vi "VolumetricFlow.vi"(9 "Pressure":dbl format="%#_13g", 10 "Tem":dbl format="%#_13g", 11 "Flow":dbl format="%#_13g") -> (3 "VolumetricFlow":dbl)   [LabVIEW 2017]
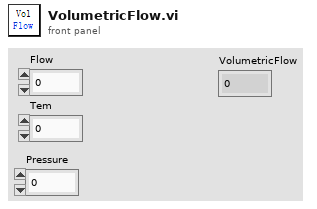
[diagram p1: front panel]
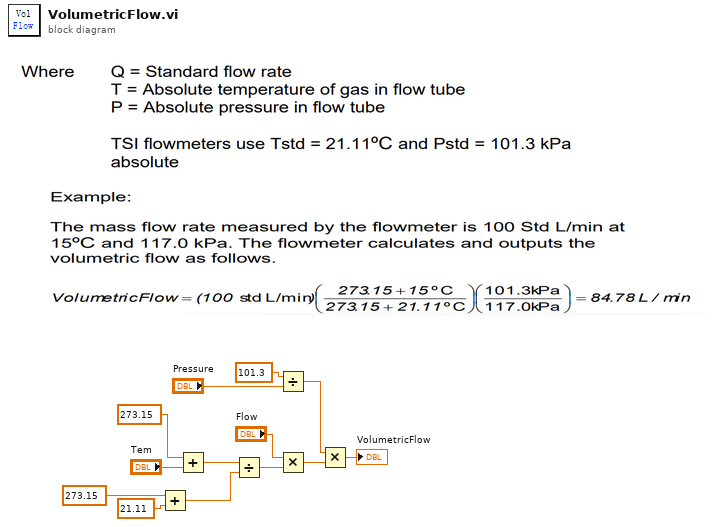
[diagram p0: block diagram]
diagram:
  n1 = Add(x=273.15, y=21.11) -> (x+y=w8:dbl)
  n2 = Add(x=273.15, y="Tem") -> (x+y=w10:dbl)
  n3 = Divide(x=w10, y=w8) -> (x/y=w6:dbl)
  n4 = Divide(x=101.3 ("y"), y="Pressure") -> (x/y=w2:dbl)
  n5 = Multiply(x="Flow", y=w6) -> (x*y=w5:dbl)
  n6 = Multiply(x=w2, y=w5) -> (x*y=→"VolumetricFlow":dbl)
